vi "Split String into Array.vi"(9 "Remove Last Row":bool, 10 "Separator":string="\n", 11 "Input string":string) -> (3 "Array of cells":string[](array[string]))   [LabVIEW 2011]
doc: "This VI splits a string copied from an Excel column into an array of cells."
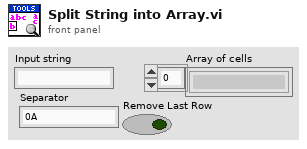
[diagram p1: front panel]
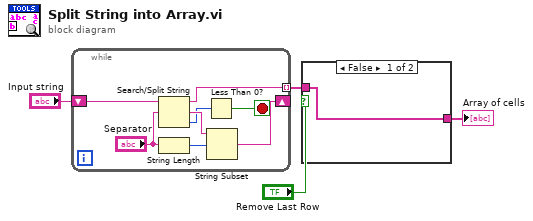
[diagram p0: block diagram]
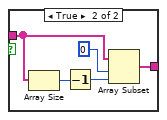
[diagram p2: hidden frame]
diagram:
  n1 = while {
    tunnel: [w8] -> w3 mode=indexing
    shift-right: [w5] -> _
    shift-left: "Input string" -> [w12]
    stop <- w6 stop-if-true
    n2 = Search/Split String(string=w12, search string/char (-)="Separator") -> (substring before match=w8:string, match + rest of string=w11:string, offset of match=w7:i32)  [unwired: 1 in]
    n3 = String Length(string="Separator") -> (length=w9:i32)
    n4 = Less Than 0?(x=w7) -> (x < 0?=w6:bool)
    n5 = String Subset(string=w11, offset (0)=w9) -> (substring=w5:string)  [unwired: 1 in]
  }
  n6 = case shown="False" "Remove Last Row" {
    tunnel: [w13 w18] -> w4
    tunnel: w3 -> [w13 w15]
    frame False {
    }
    frame True {
      n7 = Array Size(array=w15) -> (size(s)=w16:i32)
      n8 = Decrement(x=w16) -> (x-1=w17:i32)
      n9 = Array Subset(array=w15, index=0, length=w17) -> (w18:string[])
    }
  }
  "Array of cells" <- w4
